vi "test Get Attached Channels Count.vi"(11 "Test Case In":refnum<class "Test PCANBasic.lvclass">) -> (0 "error out":errorcluster, 3 "Test Case Out":refnum<class "Test PCANBasic.lvclass">)   [LabVIEW 2020, in "Test PCANBasic.lvclass"]
uses:
  Test PCANBasic.lvclass
  Test PCANBasic.lvclass/Test PCANBasic.ctl
  <vilib>/Astemes/LUnit/Test Case.lvclass
  source/PCANBasic.lvlib
  source/Get Attached Channels Count.vi
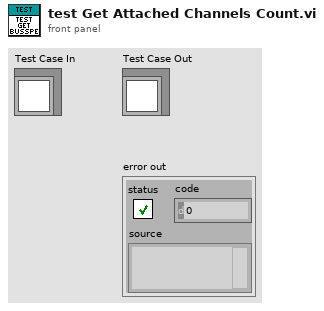
[diagram p1: front panel]
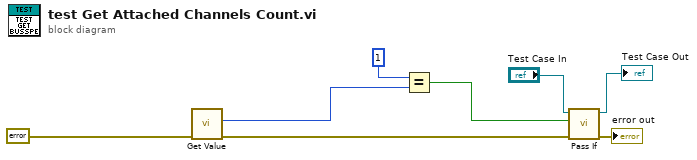
[diagram p0: block diagram]
diagram:
  n1 = call-poly "Get Value.vi"("error in"=errorcluster {"status"=FALSE, "code"=0, "source"=""}) -> ("error out"=w5:errorcluster, "Channels Count"=w2:u32)  [unwired: 8 in, 1 out]
  n2 = Equal?(x=u32 1, y=w2) -> (x = y?=w3:bool)
  n3 = call <vilib>:"Pass If.vi"("error in (no error)"=w5, "Pass?"=w3, "LUnit Test Case In"="Test Case In") -> ("error out"=→"error out":errorcluster, "LUnit Test Case Out"=→"Test Case Out":refnum<class "Test PCANBasic.lvclass">)  [unwired: 7 in]
